vi "Type String to DLL Enum.vi"(10 "Base Numeric Name":string) -> (2 "Numeric Type":T1=enum."I32")   [LabVIEW 2013, in "Number Writer.lvclass"]
doc: "Copyright (c) 2016 Sze Howe Koh\n\nThis Source Code Form is subject to the terms of the Mozilla Public License, v. 2.0. If a copy of the MPL was not distributed with this file, You can obtain one at http://mozilla.org/MPL/2.0/."
uses:
  Number Writer.lvclass
  Numeric Type.ctl
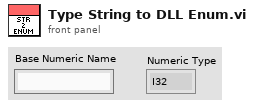
[diagram p1: front panel]
types:
  T1 = typedef "Number Writer.lvclass/Numeric Type.ctl" = enum16{"I8", "I16", "I32", "I64", "U8", "U16", "U32", "U64", "SGL", "DBL", "PTR INT", "PTR UINT"}
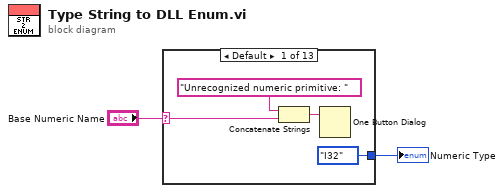
[diagram p0: block diagram]
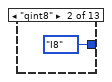
[diagram p2: hidden frame]
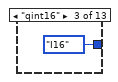
[diagram p3: hidden frame]
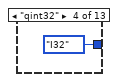
[diagram p4: hidden frame]
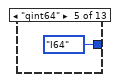
[diagram p5: hidden frame]
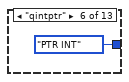
[diagram p6: hidden frame]
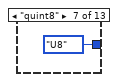
[diagram p7: hidden frame]
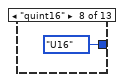
[diagram p8: hidden frame]
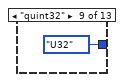
[diagram p9: hidden frame]
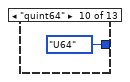
[diagram p10: hidden frame]
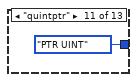
[diagram p11: hidden frame]
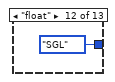
[diagram p12: hidden frame]
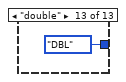
[diagram p13: hidden frame]
diagram:
  n1 = case shown="Default" "Base Numeric Name" {
    selector: "Base Numeric Name" -> [w5 _ _ _ _ _ _ _ _ _ _ _ _]
    tunnel: [Numeric_Type."I32" ("Numeric Type") Numeric_Type."I8" ("Numeric Type") Numeric_Type."I16" ("Numeric Type") Numeric_Type."I32" ("Numeric Type") Numeric_Type."I64" ("Numeric Type") Numeric_Type."PTR INT" ("Numeric Type") Numeric_Type."U8" ("Numeric Type") Numeric_Type."U16" ("Numeric Type") Numeric_Type."U32" ("Numeric Type") Numeric_Type."U64" ("Numeric Type") Numeric_Type."PTR UINT" ("Numeric Type") Numeric_Type."SGL" ("Numeric Type") Numeric_Type."DBL" ("Numeric Type")] -> w1
    frame Default {
      n2 = Concatenate Strings("Unrecognized numeric primitive: ", w5) -> (w4:string)
      n3 = One Button Dialog(message=w4) -> ()  [unwired: 1 in, 1 out]
    }
    frame "qint8" {
    }
    frame "qint16" {
    }
    frame "qint32" {
    }
    frame "qint64" {
    }
    frame "qintptr" {
    }
    frame "quint8" {
    }
    frame "quint16" {
    }
    frame "quint32" {
    }
    frame "quint64" {
    }
    frame "quintptr" {
    }
    frame "float" {
    }
    frame "double" {
    }
  }
  "Numeric Type" <- w1
